vi "New SSL Client Socket from Context.vi"(8 "error in (no error)":errorcluster, 9 "Verify hostname? (T)":bool=TRUE, 10 "Hostname / URL":string="echo.websocket.org:443", 11 "SSL Client Ctx":refnum<class "SSL Client Context.lvclass">) -> (0 "error out":errorcluster, 3 "SSL Client Skt out":refnum<class "SSL Client Socket.lvclass">)   [LabVIEW 2013, in "OpenSSL Socket.lvlib" / "SSL Client Socket.lvclass"]
doc: "Creates a new SSL Client Socket and connects to the server."
uses:
  SSL Client Socket.lvclass
  SSL Client Context/SSL Client Context.lvclass
  SSL Client Socket.lvclass/SSL Client Socket.ctl
  Write Server Hostname.vi
  Write Verify hostname.vi
  <vilib>/MediaMongrels Ltd/WebSockets/WebSockets/WebSocket Client/WebSocket Client.lvclass
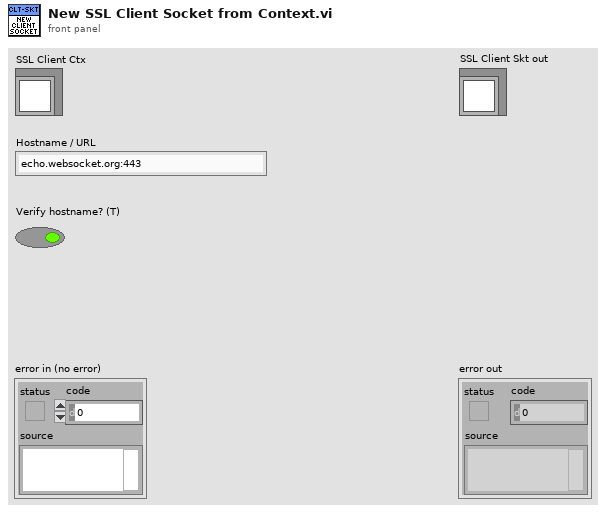
[diagram p1: front panel]
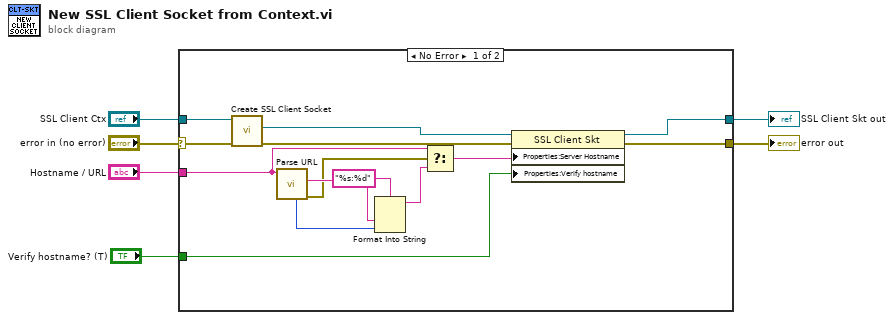
[diagram p0: block diagram]
diagram:
  n1 = case shown="No Error" "error in (no error)" {
    selector: "error in (no error)" -> [w20 w21]
    tunnel: [w13 w21] -> w5
    tunnel: "SSL Client Ctx" -> [w19 _]
    tunnel: "Hostname / URL" -> [w10 _]
    tunnel: [w12 _] -> w2
    tunnel: "Verify hostname? (T)" -> [w14 _]
    frame No Error {
      n2 = call "Create SSL Client Socket.vi"("error in (no error)"=w20, "SSL Client Ctx in"=w19) -> ("error out"=w7:errorcluster, "SSL Client Socket"=w18:refnum<class "SSL Client Socket.lvclass">)  [unwired: 7 in, 1 out]
      n3 = call <vilib>:"Parse URL.vi"("WebSocket URL"=w10) -> ("error out"=w11:errorcluster, "host"=w17:string, "port"=w16:u16)  [unwired: 6 in, 2 out]
      n4 = Format Into String(format string="%s:%d", w17, w16) -> (resulting string=w9:string)  [unwired: 2 in, 1 out]
      n5 = Select(t=w10, s=w11, f=w9) -> (s? t:f=w8:string)
      n6 = property class="SSL Client Skt"(reference=w18, error in=w7, "Properties:Server Hostname"=w8, "Properties:Verify hostname"=w14) -> (reference out=w12:refnum<class "SSL Client Socket.lvclass">, error out=w13:errorcluster)
    }
    frame Error {
    }
  }
  "error out" <- w5
  "SSL Client Skt out" <- w2
